vi "DefaultFromIni.vi"(8 "error in (no error)":errorcluster, 11 "SpecAnPlugins.lvlib":refnum<class "SpecAnBase.lvclass">) -> (0 "error out":errorcluster, 3 "SpecAnPlugins.lvlib":refnum<class "SpecAnBase.lvclass">)   [LabVIEW 2018, in "SpecAnPlugins.lvlib" / "SpecAnBase.lvclass"]
doc: "This VI loads the configuration previously stored into memory for future acquisitions and generations"
uses:
  SpecAnBase.lvclass
  C:/Program Files (x86)/National Instruments/LabVIEW 2018/user.lib/NIST/BaseClasses/BasePlugin_class/BasePlugin.lvclass
  Typedefs/Acquisition.ctl
  Typedefs/Frequency.ctl
  Typedefs/Level.ctl
  Typedefs/SweepCoupling.ctl
  Typedefs/Trace.ctl
  Typedefs/Trigger.ctl
  <userlib>/NIST/BaseClasses/BasePlugin_class/BasePlugin.lvclass/BasePlugin.ctl
  <userlib>/NIST/BaseClasses/BasePlugin_class/Accessors/Read PluginIniFilePath.vi
  <vilib>/Utility/config.llb/NI_LVConfig.lvlib
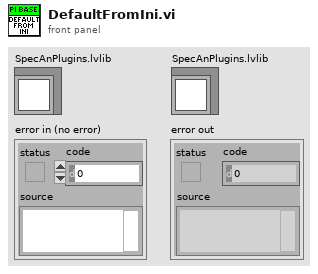
[diagram p1: front panel]
types:
  T1 = typedef "SpecAnPlugins.lvlib/SpecAnBase.lvclass/Trigger.ctl" = cluster{"TriggerLevel":dbl, "TriggerSlope":i32, "Trigger Source":i32}
  T2 = typedef "SpecAnPlugins.lvlib/SpecAnBase.lvclass/Trace.ctl" = cluster{"TraceName":string, "TraceSize":i32, "TraceType":i32}[]
  T3 = typedef "SpecAnPlugins.lvlib/SpecAnBase.lvclass/SweepCoupling.ctl" = cluster{"ResolutionBandwidth":dbl, "ResolutionBandwidthAuto":bool, "SweepTime":dbl, "VideoBandwidth":dbl, "VideoBandwidthAuto":bool, "SweepTimeAuto":bool}
  T4 = typedef "SpecAnPlugins.lvlib/SpecAnBase.lvclass/Level.ctl" = cluster{"InputImpedance":dbl, "AttenuationAuto":bool, "ReferenceLevel":dbl, "Attenuation":dbl, "ReferenceLevelOffset":dbl, "amplitude units (dBm)":i32}
  T5 = typedef "SpecAnPlugins.lvlib/SpecAnBase.lvclass/Frequency.ctl" = cluster{"FrequencyStart":dbl, "FrequencyStop":dbl, "FrequencyOffset":dbl}
  T6 = typedef "SpecAnPlugins.lvlib/SpecAnBase.lvclass/Acquisition.ctl" = cluster{"Handle":string, "Connected":bool, "Enabled":bool, "SweepModeContinuous":bool, "NumberOfSweeps":i32, "DetectorTypeAuto":bool, "DetectorType":i32, "VerticalScale":i32, "MaximumTime(seconds)":dbl}
  T7 = typedef "NI_LVConfig.lvlib/Config Data RefNum.ctl" = refnum<k1>
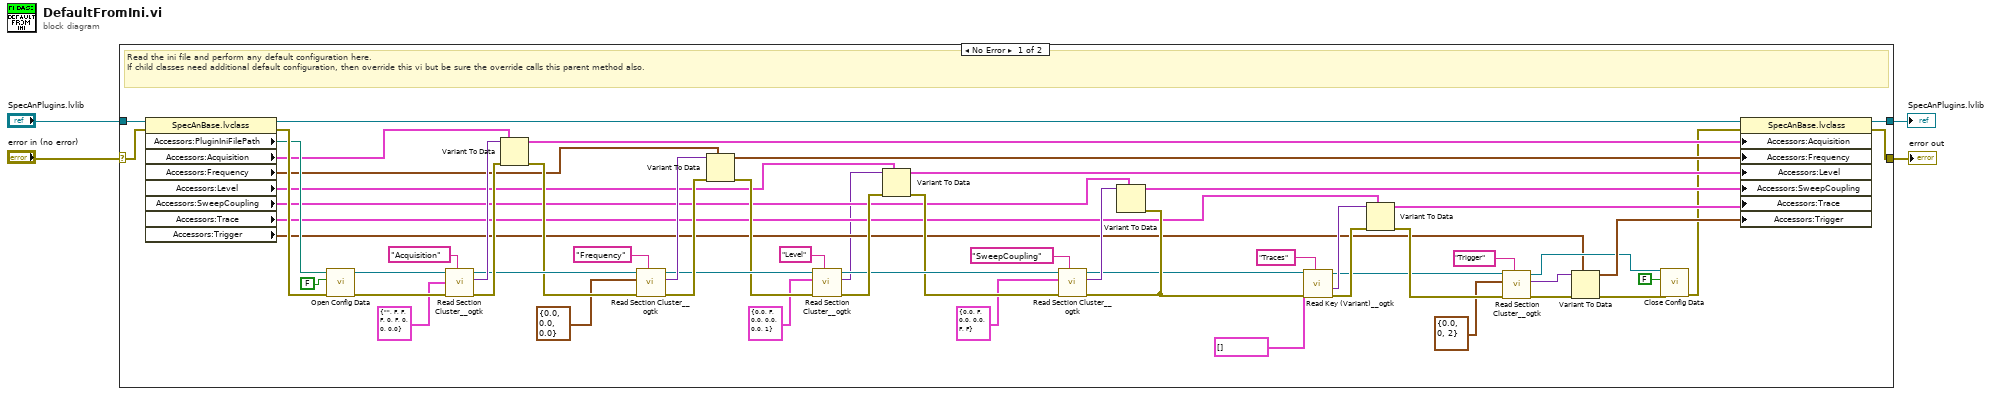
[diagram p0: block diagram]
diagram:
  n1 = case shown="No Error" "error in (no error)" {
    selector: "error in (no error)" -> [w62 w65]
    tunnel: [w59 w65] -> w3
    tunnel: [w60 w64] -> w1
    tunnel: "SpecAnPlugins.lvlib" -> [w63 w64]
    frame No Error {
      # "Read the ini file and perform any default configuration here.\nIf child classes need additional default configuration, then override this vi but be sure the override calls this parent method also."
      n2 = property class="SpecAnBase.lvclass"(reference=w63, error in=w62) -> (reference out=w61:refnum<class "SpecAnBase.lvclass">, error out=w57:errorcluster, "Accessors:PluginIniFilePath"=w56:path, "Accessors:Acquisition"=w18:T6, "Accessors:Frequency"=w17:T5, "Accessors:Level"=w16:T4, "Accessors:SweepCoupling"=w15:T3, "Accessors:Trace"=w14:T2, "Accessors:Trigger"=w13:T1)
      n3 = call <vilib>:"Open Config Data.vi"("error in (no error)"=w57, "create file if necessary (T)"=FALSE, "configuration file path"=w56) -> ("error out"=w55:errorcluster, "refnum"=w54:T7)  [unwired: 6 in, 1 out]
      n4 = call <userlib>:"Read Section Cluster__ogtk.vi"("section (optional)"="Acquisition", "error in (no error)"=w55, "Section Formatted Cluster Type"=T6 {"Handle"="", "Connected"=FALSE, "Enabled"=FALSE, "SweepModeContinuous"=FALSE, "NumberOfSweeps"=0, "DetectorTypeAuto"=FALSE, "DetectorType"=0, "VerticalScale"=0, "MaximumTime(seconds)"=0.0} ("Acquisition"), "refnum"=w54) -> ("error out"=w51:errorcluster, "Section Formatted Cluster"=w52:variant, "dup refnum"=w50:T7)  [unwired: 3 in, 2 out]
      n5 = Variant To Data(error in=w51, type=w18, Variant=w52) -> (data=w46:T6, error out=w49:errorcluster)
      n6 = call <userlib>:"Read Section Cluster__ogtk.vi"("section (optional)"="Frequency", "error in (no error)"=w49, "Section Formatted Cluster Type"=T5 {"FrequencyStart"=0.0, "FrequencyStop"=0.0, "FrequencyOffset"=0.0} ("Frequency"), "refnum"=w50) -> ("error out"=w48:errorcluster, "Section Formatted Cluster"=w47:variant, "dup refnum"=w41:T7)  [unwired: 3 in, 2 out]
      n7 = Variant To Data(error in=w48, type=w17, Variant=w47) -> (data=w44:T5, error out=w40:errorcluster)
      n8 = call <userlib>:"Read Section Cluster__ogtk.vi"("section (optional)"="Level", "error in (no error)"=w40, "Section Formatted Cluster Type"=T4 {"InputImpedance"=0.0, "AttenuationAuto"=FALSE, "ReferenceLevel"=0.0, "Attenuation"=0.0, "ReferenceLevelOffset"=0.0, "amplitude units (dBm)"=1} ("Level"), "refnum"=w41) -> ("error out"=w42:errorcluster, "Section Formatted Cluster"=w11:variant, "dup refnum"=w36:T7)  [unwired: 3 in, 2 out]
      n9 = Variant To Data(error in=w42, type=w16, Variant=w11) -> (data=w39:T4, error out=w35:errorcluster)
      n10 = call <userlib>:"Read Section Cluster__ogtk.vi"("section (optional)"="SweepCoupling", "error in (no error)"=w35, "Section Formatted Cluster Type"=T3 {"ResolutionBandwidth"=0.0, "ResolutionBandwidthAuto"=FALSE, "SweepTime"=0.0, "VideoBandwidth"=0.0, "VideoBandwidthAuto"=FALSE, "SweepTimeAuto"=FALSE} ("SweepCoupling"), "refnum"=w36) -> ("error out"=w32:errorcluster, "Section Formatted Cluster"=w38:variant, "dup refnum"=w24:T7)  [unwired: 3 in, 2 out]
      n11 = Variant To Data(error in=w32, type=w15, Variant=w38) -> (data=w31:T3)  [unwired: 1 out]
      n12 = call <userlib>:"Read Key (Variant)__ogtk.vi"("section"="Traces" ("section (optional)"), "error in (no error)"=w32, "type"=T2 [] ("Trace"), "refnum"=w24) -> ("error out"=w33:errorcluster, "key-value"=w34:variant, "refnum out"=w23:T7)  [unwired: 4 in, 1 out]
      n13 = Variant To Data(error in=w33, type=w14, Variant=w34) -> (data=w30:T2, error out=w26:errorcluster)
      n14 = call <userlib>:"Read Section Cluster__ogtk.vi"("section (optional)"="Trigger", "error in (no error)"=w26, "Section Formatted Cluster Type"=T1 {"TriggerLevel"=0.0, "TriggerSlope"=0, "Trigger Source"=2} ("Trigger"), "refnum"=w23) -> ("error out"=w29:errorcluster, "Section Formatted Cluster"=w28:variant, "dup refnum"=w20:T7)  [unwired: 3 in, 2 out]
      n15 = Variant To Data(error in=w29, type=w13, Variant=w28) -> (data=w25:T1, error out=w22:errorcluster)
      n16 = call <vilib>:"Close Config Data.vi"("error in (no error)"=w22, "write file if changed (T)"=FALSE, "refnum"=w20) -> ("error out"=w21:errorcluster)  [unwired: 7 in, 1 out]
      n17 = property class="SpecAnBase.lvclass"(reference=w61, error in=w21, "Accessors:Acquisition"=w46, "Accessors:Frequency"=w44, "Accessors:Level"=w39, "Accessors:SweepCoupling"=w31, "Accessors:Trace"=w30, "Accessors:Trigger"=w25) -> (reference out=w60:refnum<class "SpecAnBase.lvclass">, error out=w59:errorcluster)
    }
    frame Error {
    }
  }
  "error out" <- w3
  "SpecAnPlugins.lvlib" <- w1
